vi "2D_TO_1D_P.vi"(9 "indice colonne courant":i32, 11 "Array 2D":dbl[][](array[numeric])) -> (2 "Array1D size":i32, 3 "Array 1D":dbl[](array[numeric]))   [LabVIEW 2020]
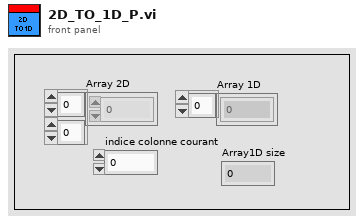
[diagram p1: front panel]
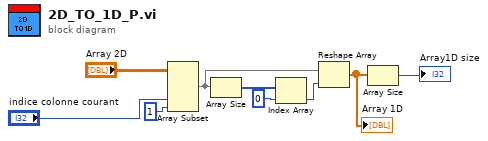
[diagram p0: block diagram]
diagram:
  n1 = Array Subset(array="Array 2D", index (col)="indice colonne courant", length (col)=1 ("length")) -> (w8:dbl[][])  [unwired: 2 in]
  n2 = Array Size(array=w8) -> (size(s)=w6:i32[])
  n3 = Index Array(array=w6, index=0) -> (element=w4:i32)
  n4 = Reshape Array(w8, w4) -> (w3:dbl[])
  "Array 1D" <- w3
  n5 = Array Size(array=w3) -> (size(s)=→"Array1D size":i32)
